vi "打包数据.vi"(1 "补充信息":string[](array[string]), 2 "备选信息":string[](array[string])) -> (0 "语句":string)   [LabVIEW 2020]
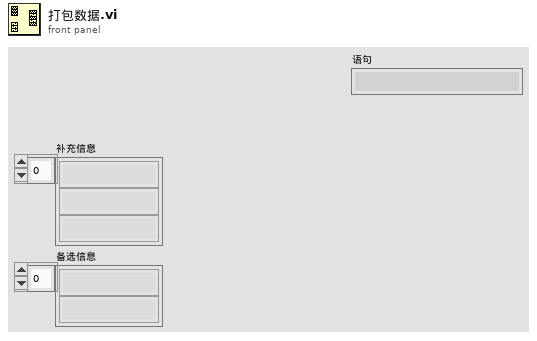
[diagram p1: front panel]
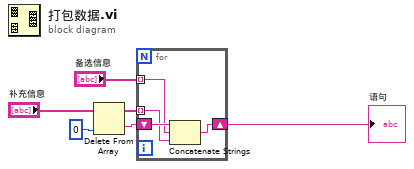
[diagram p0: block diagram]
diagram:
  n1 = Delete From Array(array="补充信息", index=0 ("索引")) -> (deleted portion=w2:string, array with subset deleted=w4:string[])  [unwired: 1 in]
  n2 = for {
    tunnel: "备选信息" -> [w8] mode=indexing
    tunnel: w4 -> [w7] mode=indexing
    shift-right: [w9] -> w1
    shift-left: w2 -> [w10]
    n3 = Concatenate Strings(w10, w8, w7) -> (w9:string)
  }
  "语句" <- w1
